vi "CalibComputeRatio.vi"(8 "error in (no error)":errorcluster, 11 "Desired Refresh Ratio":dbl) -> (0 "error out":errorcluster, 3 "Pump steps for the\n desired refresh ratio":dbl)   [LabVIEW 2018]
panel:
  in  "Calib Image File":path
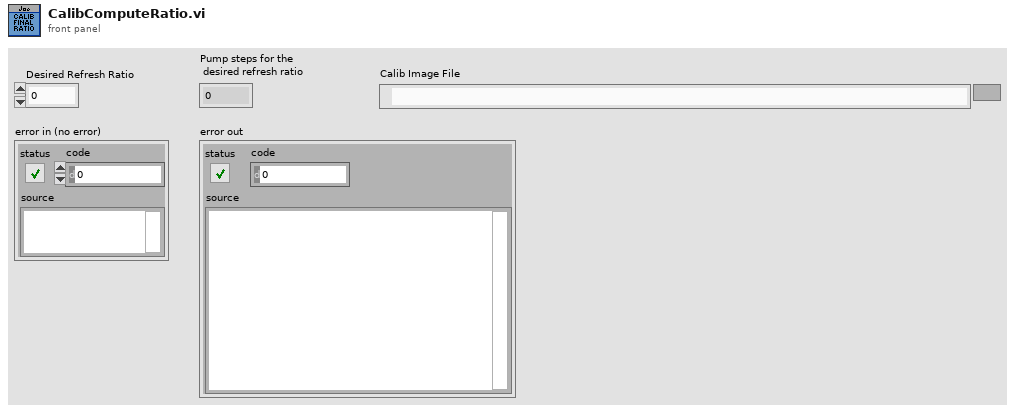
[diagram p1: front panel]
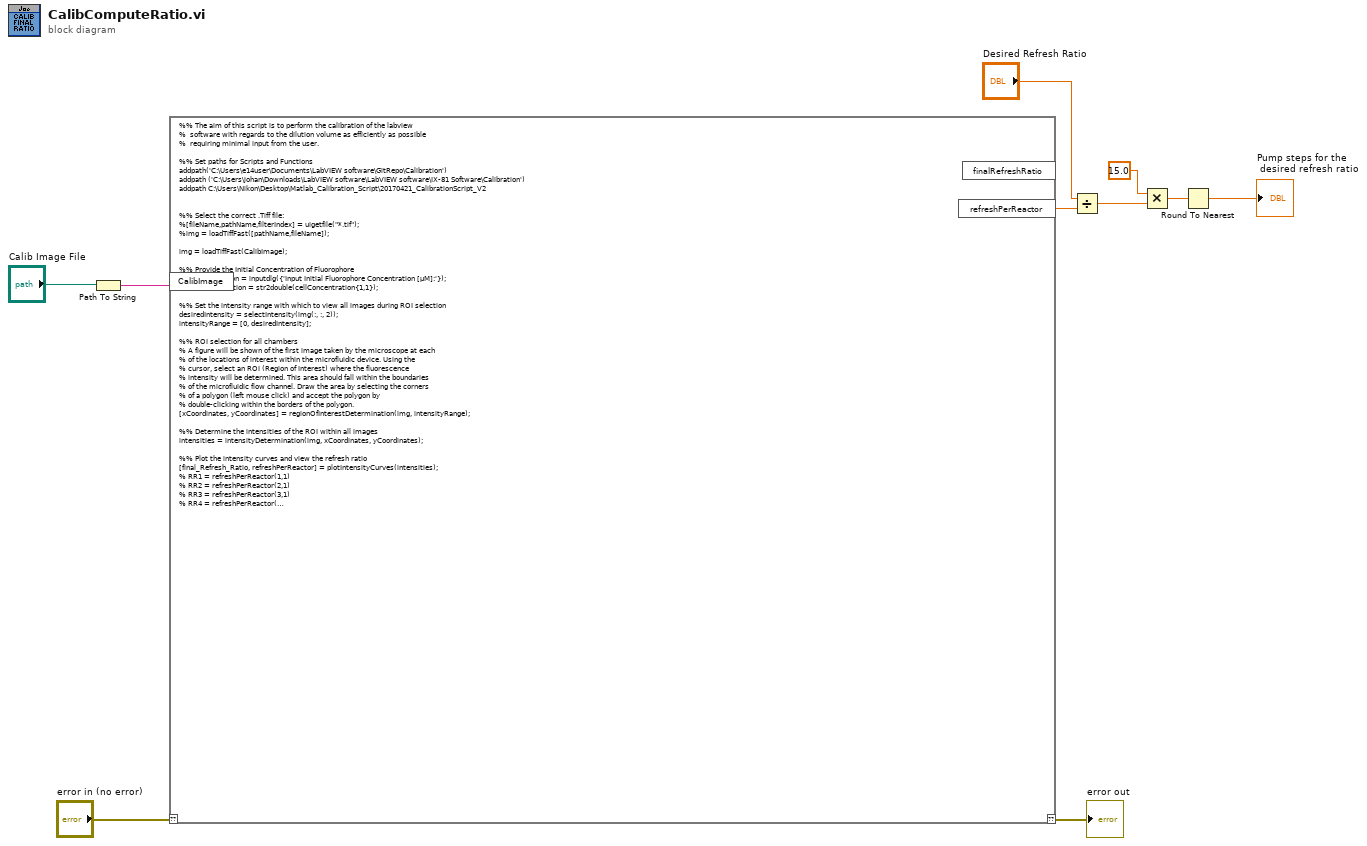
[diagram p0: block diagram]
diagram:
  n1 = Path To String(path="Calib Image File") -> (string=w1:string)
  n2 = script code="%% The aim of this script is to perform the calibration of the labview\n%  software with regards to the dilution volume as efficiently as possible\n%  requiring minimal input from the user. \n\n%% Set paths for Scripts and Functions\naddpath('C:\\Users\\e14user\\Documents\\LabVIEW software\\GitRepo\\Calibration')\naddpath ('C:\\Users\\johan\\Downloads\\LabVIEW software\\LabVIEW software\\IX-81 Software\\Calibration')\naddpath C:\\Users\\Nikon\\Desktop\\Matlab_Calibration_Script\\20170421_CalibrationScript_V2\n\n\n%% Select the correct .Tiff file:\n%[fileName,pathName,filterIndex] = uigetfile(\"*.tif\");\n%img = loadTiffFast([pathName,fileName]);\n\nimg = loadTiffFast(CalibImage);\n\n%% Provide the Initial Concentration of Fluorophore\ncellConcentration = inputdlg({'Input Initial Fluorophore Concentration [µM]:'});\ninitialConcentration = str2double(cellConcentration{1,1});\n\n%% Set the intensity range with which to view all images during ROI selection\ndesiredIntensity = selectIntensity(img(:, :, 2));\nintensityRange = [0, desiredIntensity];\n\n%% ROI selection for all chambers\n% A figure will be shown of the first image taken by the microscope at each\n% of the locations of interest within the microfluidic device. Using the\n% cursor, select an ROI (Region of Interest) where the fluorescence\n% intensity will be determined. This area should fall within the boundaries\n% of the microfluidic flow channel. Draw the area by selecting the corners\n% of a polygon (left mouse click) and accept the polygon by\n% double-clicking within the borders of the polygon. \n[xCoordinates, yCoordinates] = regionOfInterestDetermination(img, intensityRange);\n\n%% Determine the intensities of the ROI within all images\nintensities = intensityDetermination(img, xCoordinates, yCoordinates);\n\n%% Plot the intensity curves and view the refresh ratio\n[final_Refresh_Ratio, refreshPerReactor] = plotIntensityCurves(intensities);\n% RR1 = refreshPerReactor(1,1)\n% RR2 = refreshPerReactor(2,1)\n% RR3 = refreshPerReactor(3,1)\n% RR4 = refreshPerReactor(4,1)\n% RR5 = refreshPerReactor(5,1)\n% RR6 = refreshPerReactor(6,1)\n% RR7 = refreshPerReactor(7,1)\n% RR8 = refreshPerReactor(8,1)\n\n%% This is the end of the script."("??"="error in (no error)", "CalibImage"=w1) -> ("??"=→"error out":errorcluster, "refreshPerReactor"=w7:dbl)  [unwired: 1 out]
  n3 = Divide(x="Desired Refresh Ratio", y=w7) -> (x/y=w5:dbl)
  n4 = Multiply(x=15.0, y=w5) -> (x*y=w6:dbl)
  n5 = Round To Nearest(number=w6) -> (nearest integer value=→"Pump steps for the\n desired refresh ratio":dbl)
